vi "File.Get File List based on Pattern, Check SubDirs.vi"(9 "Max Files":i32=2, 10 "Pattern":string="*Data.csv", 11 "Dirs":path[](array[path])) -> (3 "Files":path[](array[path]))   [LabVIEW 2019]
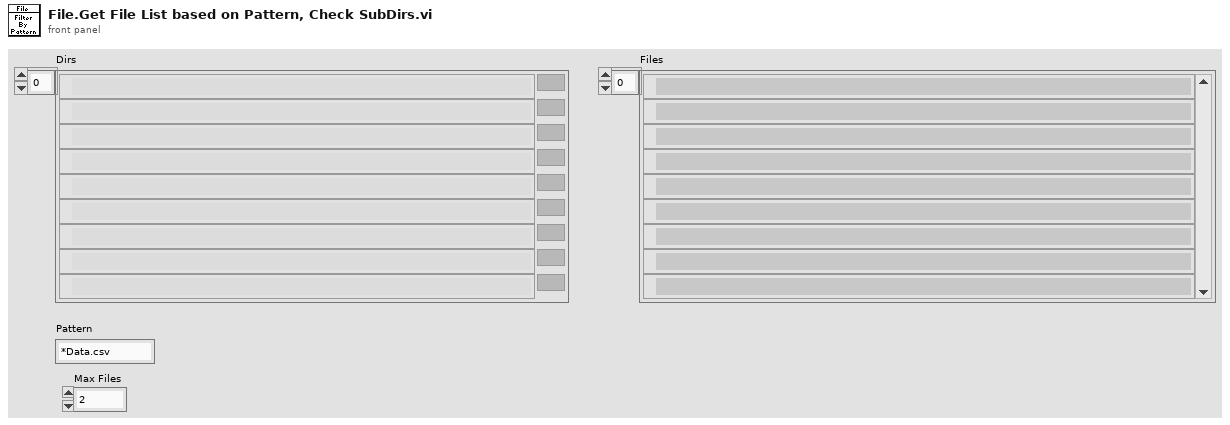
[diagram p1: front panel]
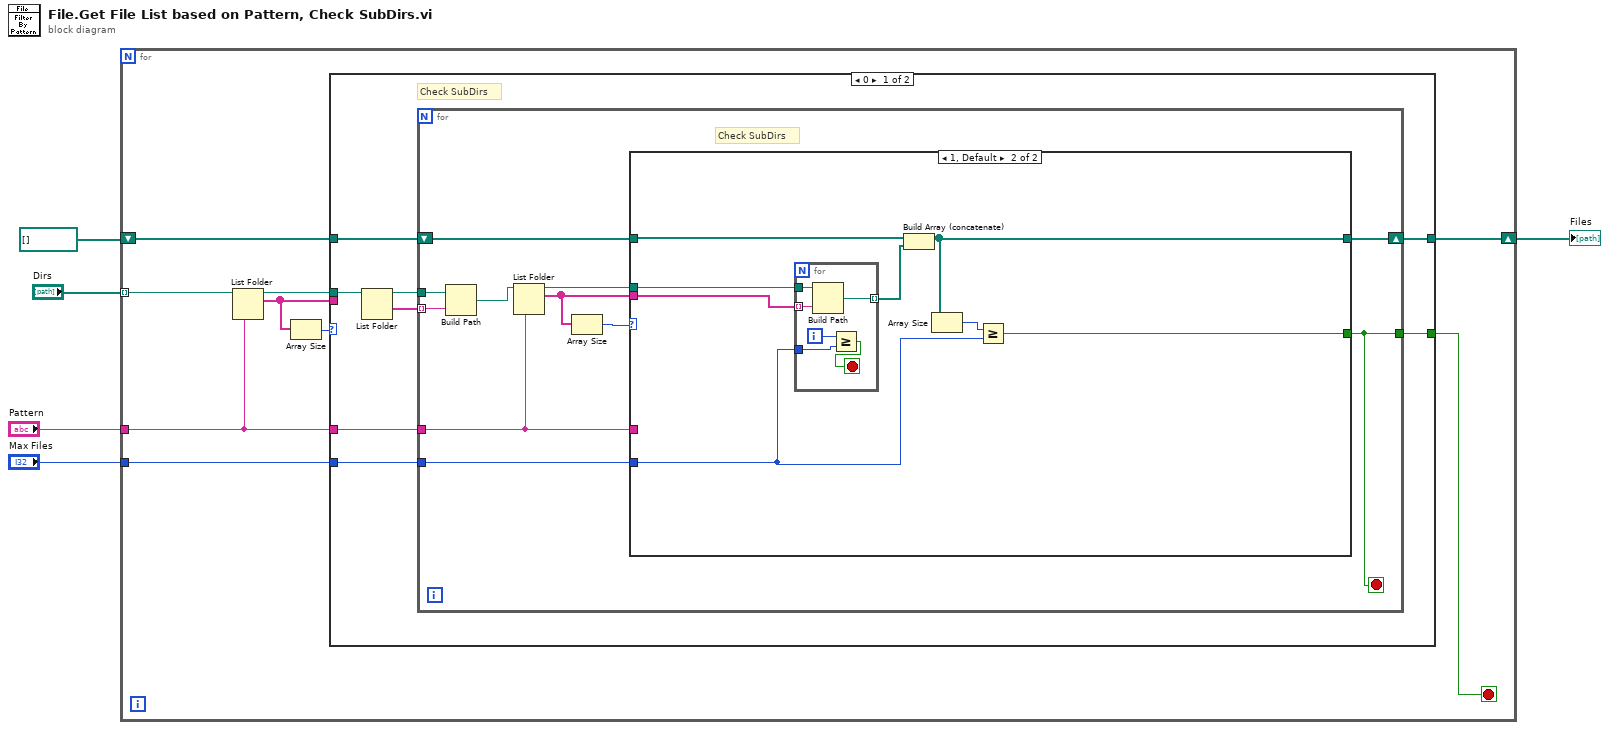
[diagram p0: block diagram]
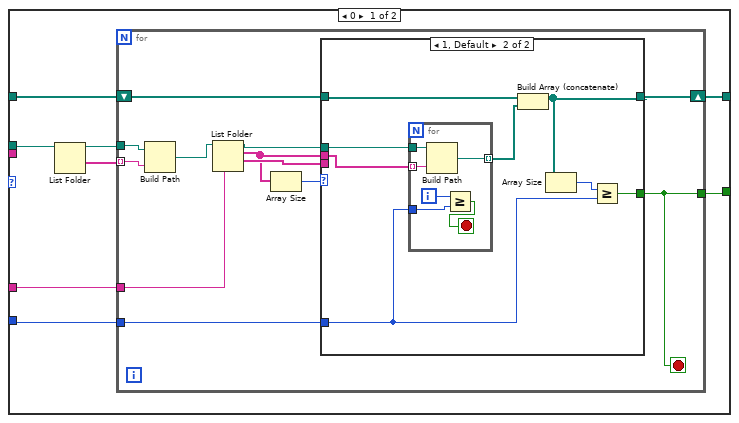
[diagram p2: hidden frame]
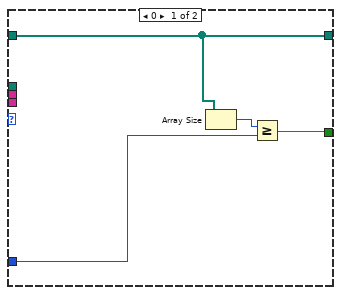
[diagram p3: hidden frame]
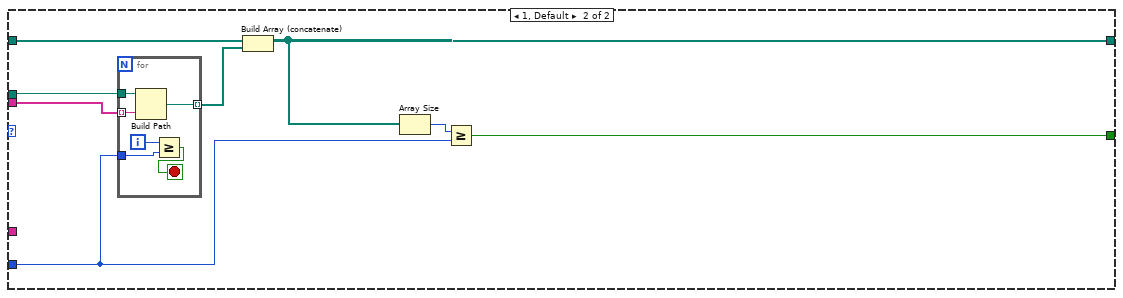
[diagram p4: hidden frame]
diagram:
  n1 = for {
    tunnel: "Dirs" -> [w13] mode=indexing
    tunnel: "Pattern" -> [w6]
    shift-right: [w9] -> w2
    shift-left: path[] [] ("Files") -> [w10]
    tunnel: "Max Files" -> [w8]
    stop <- w7 stop-if-true
    n2 = List Folder(path=w13, pattern=w6) -> (path out=w14:path, filenames=w11:string[])  [unwired: 2 in, 2 out]
    n3 = Array Size(array=w11) -> (size(s)=w12:i32)
    n4 = case shown="0" w12 {
      tunnel: w14 -> [w17 w92]
      tunnel: w11 -> [_ w91]
      tunnel: w10 -> [w20 w93]
      tunnel: [w19 w89] -> w9
      tunnel: w8 -> [w21 w87]
      tunnel: [w18 w86] -> w7
      tunnel: w6 -> [w22 _]
      frame 0 {
        # "Check SubDirs"
        n5 = List Folder(path=w17) -> (path out=w16:path, folder names=w15:string[])  [unwired: 3 in, 2 out]
        n6 = for {
          tunnel: w16 -> [w33]
          tunnel: w15 -> [w32] mode=indexing
          tunnel: w22 -> [w26]
          tunnel: w21 -> [w27]
          shift-right: [w24] -> w19
          shift-left: w20 -> [w25]
          tunnel: [w23] -> w18
          stop <- w23 stop-if-true
          # "Check SubDirs"
          n7 = Build Path(base path=w33, name or relative path=w32) -> (appended path=w31:path)
          n8 = List Folder(path=w31, pattern=w26) -> (path out=w30:path, filenames=w29:string[])  [unwired: 2 in, 2 out]
          n9 = Array Size(array=w29) -> (size(s)=w28:i32)
          n10 = case shown="1, Default" w28 {
            tunnel: w30 -> [w36 w76]
            tunnel: w29 -> [_ w75]
            tunnel: w27 -> [w38 w74]
            tunnel: w26 -> [w41 _]
            tunnel: w25 -> [w40 w77]
            tunnel: [w39 w73] -> w24
            tunnel: [w37 w72] -> w23
            frame 0 {
              n11 = List Folder(path=w36) -> (path out=w35:path, folder names=w34:string[])  [unwired: 3 in, 2 out]
              n12 = for {
                tunnel: w35 -> [w52]
                tunnel: w34 -> [w51] mode=indexing
                tunnel: w41 -> [w50]
                shift-right: [w48] -> w39
                shift-left: w40 -> [w49]
                tunnel: w38 -> [w43]
                tunnel: [w42] -> w37
                stop <- w42 stop-if-true
                n13 = Build Path(base path=w52, name or relative path=w51) -> (appended path=w53:path)
                n14 = List Folder(path=w53, pattern=w50) -> (path out=w46:path, filenames=w44:string[], folder names=w45:string[])  [unwired: 2 in, 1 out]
                n15 = Array Size(array=w44) -> (size(s)=w47:i32)
                n16 = case shown="1, Default" w47 {
                  tunnel: w49 -> [w56 w63]
                  tunnel: [w56 w62] -> w48
                  tunnel: w46 -> [_ w61]
                  tunnel: w45 -> [_ _]
                  tunnel: w44 -> [_ w60]
                  tunnel: w43 -> [w55 w59]
                  tunnel: [w54 w58] -> w42
                  frame 0 {
                    n17 = Array Size(array=w56) -> (size(s)=w57:i32)
                    n18 = Greater Or Equal?(x=w57, y=w55) -> (x >= y?=w54:bool)
                  }
                  frame 1, Default {
                    n19 = for {
                      tunnel: w61 -> [w71]
                      tunnel: w60 -> [w70] mode=indexing
                      tunnel: [w69] -> w65 mode=indexing
                      tunnel: w59 -> [w67]
                      i -> [w68]
                      stop <- w66 stop-if-true
                      n20 = Build Path(base path=w71, name or relative path=w70) -> (appended path=w69:path)
                      n21 = Greater Or Equal?(x=w68, y=w67) -> (x >= y?=w66:bool)
                    }
                    n22 = Build Array (concatenate)(w63, w65) -> (w62:path[])
                    n23 = Array Size(array=w62) -> (size(s)=w64:i32)
                    n24 = Greater Or Equal?(x=w64, y=w59) -> (x >= y?=w58:bool)
                  }
                }
              }
            }
            frame 1, Default {
              n25 = for {
                tunnel: w76 -> [w85]
                tunnel: w75 -> [w84] mode=indexing
                tunnel: [w83] -> w79 mode=indexing
                tunnel: w74 -> [w81]
                i -> [w82]
                stop <- w80 stop-if-true
                n26 = Build Path(base path=w85, name or relative path=w84) -> (appended path=w83:path)
                n27 = Greater Or Equal?(x=w82, y=w81) -> (x >= y?=w80:bool)
              }
              n28 = Build Array (concatenate)(w77, w79) -> (w73:path[])
              n29 = Array Size(array=w73) -> (size(s)=w78:i32)
              n30 = Greater Or Equal?(x=w78, y=w74) -> (x >= y?=w72:bool)
            }
          }
        }
      }
      frame 1, Default {
        n31 = for {
          tunnel: w92 -> [w99]
          tunnel: w91 -> [w98] mode=indexing
          tunnel: [w97] -> w90 mode=indexing
          tunnel: w87 -> [w95]
          i -> [w96]
          stop <- w94 stop-if-true
          n32 = Build Path(base path=w99, name or relative path=w98) -> (appended path=w97:path)
          n33 = Greater Or Equal?(x=w96, y=w95) -> (x >= y?=w94:bool)
        }
        n34 = Build Array (concatenate)(w93, w90) -> (w89:path[])
        n35 = Array Size(array=w89) -> (size(s)=w88:i32)
        n36 = Greater Or Equal?(x=w88, y=w87) -> (x >= y?=w86:bool)
      }
    }
  }
  "Files" <- w2
